vi "4.Light sensor_0.vi"() -> ()   [LabVIEW 2015]
uses:
  <vilib>/myRIO/Instrument Drivers/Onboard IO/DIO/vis/Write.vi
  <vilib>/myRIO/Instrument Drivers/Onboard IO/SPI/vis/Configure.vi
  <vilib>/myRIO/Instrument Drivers/Onboard IO/SPI/vis/Read.vi
  <vilib>/myRIO/Common/Instrument Driver Framework/myRIO v1.0/UART/vis/myRIO v1.0 Close UART.vi
  <vilib>/myRIO/Instrument Drivers/Onboard IO/SPI/vis/Write Read.vi
  <vilib>/myRIO/Instrument Drivers/Onboard IO/DIO/vis/Smart Open.vi
  <vilib>/Utility/error.llb/Error Cluster From Error Code.vi
  <vilib>/myRIO/Common/Instrument Driver Framework/myRIO v1.0/DIO/vis/myRIO v1.0 Write DIO.vi
  <vilib>/myRIO/Instrument Drivers/Onboard IO/SPI/vis/Smart Open.vi
  <vilib>/myRIO/Common/Instrument Driver Framework/myRIO v1.0/SPI/vis/myRIO v1.0 Configure SPI.vi
  <vilib>/myRIO/Common/Instrument Driver Framework/myRIO v1.0/SPI/vis/myRIO v1.0 Write Read SPI.vi
  <vilib>/myRIO/Common/Instrument Driver Framework/Utilities/vis/FPGA Ref Manager.vi
  <vilib>/myRIO/Common/Instrument Driver Framework/myRIO v1.0/myRIO v1.0 Reset FPGA.vi
  <vilib>/myRIO/Common/Instrument Driver Framework/myRIO v1.0/IRQ/vis/myRIO v1.0 IRQ Info FGV.vi
  <vilib>/myRIO/Common/Instrument Driver Framework/myRIO v1.0/IRQ/vis/myRIO v1.0 Timer IRQ Info FGV.vi
  <vilib>/myRIO/Common/Instrument Driver Framework/myRIO v1.0/IRQ/vis/myRIO v1.0 ISR Agent.vi
  <vilib>/myRIO/Instrument Drivers/Utilities/Utilities.lvlib
panel:
  in  "Tab Control":enum32{"Page 1", "Page 2"}(tab)
  in  "[ESC]":bool
  out "sensor value":u8(knob) scale=0.0..255.0
  # "Ambient Light Sensor demo"
  # "Pardeep kumar"
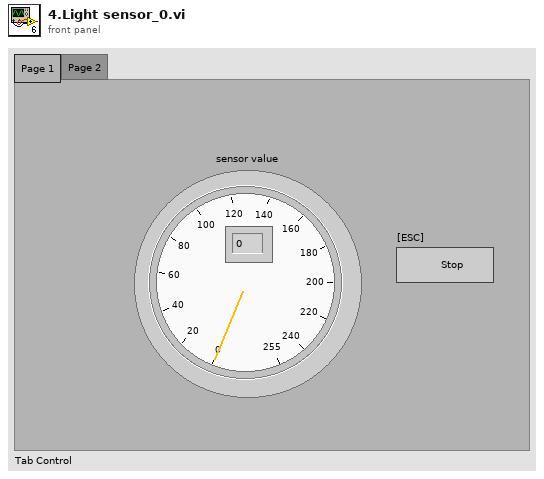
[diagram p1: front panel]
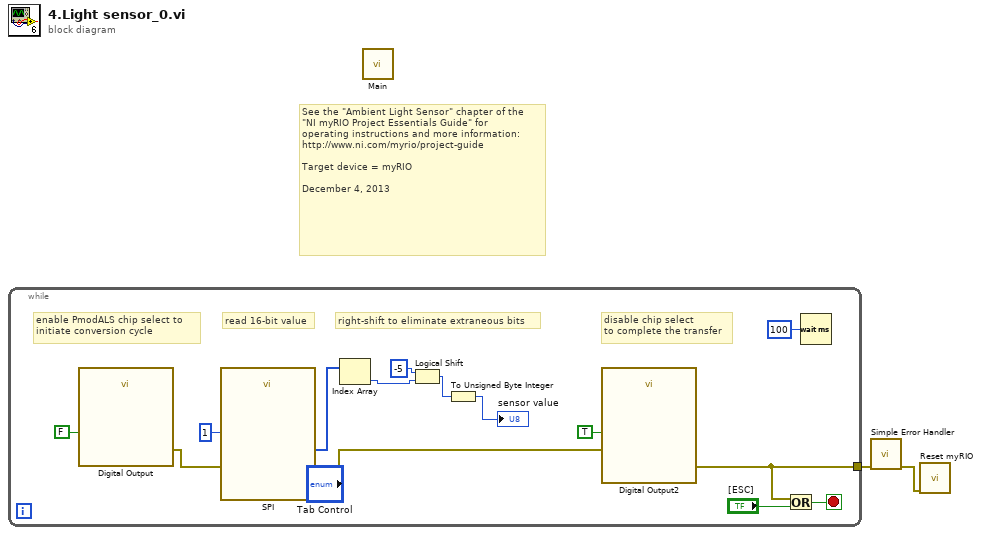
[diagram p0: block diagram]
diagram:
  # "See the \"Ambient Light Sensor\" chapter of the\n\"NI myRIO Project Essentials Guide\" for\noperating instructions and more information: \nhttp://www.ni.com/myrio/project-guide\n\nTarget device = myRIO\n\nDecember 4, 2013"
  n1 = while {
    tunnel: [w9] -> w2
    stop <- w16 stop-if-true
    # "right-shift to eliminate extraneous bits"
    # "disable chip select\nto complete the transfer"
    # "read 16-bit value"
    # "enable PmodALS chip select to\ninitiate conversion cycle"
    n2 = call "Digital Output"("B/DIO0 (Pin 11)"=FALSE ("A/DIO0 (Pin 11)")) -> ("error out"=w12:errorcluster)  [unwired: 26 in]
    n3 = call "SPI"("Frame Count"=u32 1, "error in (no error)"=w12) -> ("Frames Read"=w7:u16[], "error out"=w10:errorcluster)  [unwired: 24 in]
    n4 = Index Array "Index Array"(array=w7) -> (element=w6:u16)  [unwired: 1 in]
    n5 = Logical Shift(y=i16 -5, x=w6) -> (x << y=w4:u16)
    n6 = To Unsigned Byte Integer(number=w4) -> (unsigned 8bit integer=→"sensor value":u8)
    n7 = call "Digital Output2"("B/DIO0 (Pin 11)"=TRUE ("A/DIO0 (Pin 11)"), "error in (no error)"=w10) -> ("error out"=w9:errorcluster)  [unwired: 25 in]
    n8 = Or(x=w9, y="[ESC]") -> (x .or. y?=w16:bool)
    n9 = Wait (ms)(milliseconds to wait=u32 100) -> ()  [unwired: 1 out]
  }
  n10 = call "Main.vi"() -> ()  [unwired: 12 in]
  n11 = call <vilib>:"Simple Error Handler.vi"("error in (no error)"=w2) -> ("error out"=w1:errorcluster)  [unwired: 4 in, 4 out]
  n12 = call <vilib>:"Reset myRIO.vi"("error in (no error)"=w1) -> ()  [unwired: 10 in, 1 out]
